vi "Angle Loop.vi"(1 "Input Angle":dbl format="%#_13g") -> (0 "Output Angle":dbl)   [LabVIEW 2018]
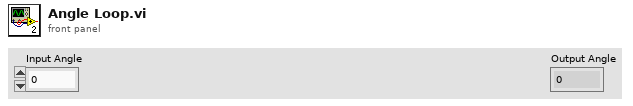
[diagram p1: front panel]
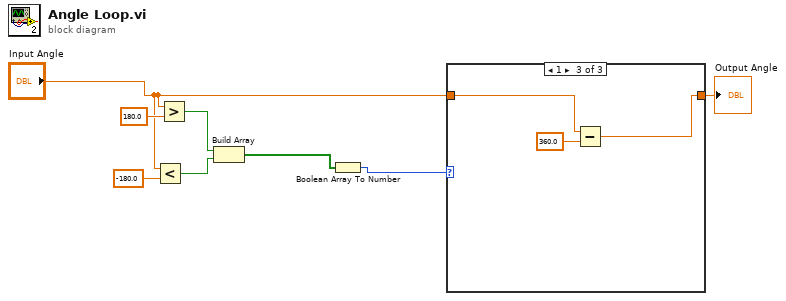
[diagram p0: block diagram]
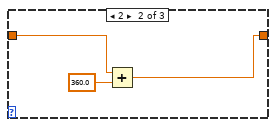
[diagram p3: hidden frame]
diagram:
  n1 = Less?(x="Input Angle", y=-180.0) -> (x < y?=w7:bool)
  n2 = Greater?(x="Input Angle", y=180.0) -> (0:w8:bool)
  n3 = Build Array(w8, w7) -> (w6:bool[])
  n4 = Boolean Array To Number(Boolean array=w6) -> (number=w5:u32)
  n5 = case shown="1" w5 {
    tunnel: "Input Angle" -> [w9 w11 w14]
    tunnel: [w9 w12 w15] -> w1
    frame 0, Default {
    }
    frame 2 {
      n6 = Add(x=w11, y=360.0) -> (x+y=w12:dbl)
    }
    frame 1 {
      n7 = Subtract(x=w14, y=360.0) -> (x-y=w15:dbl)
    }
  }
  "Output Angle" <- w1
